vi "WriteINI.vi"(8 "Error In":errorcluster, 11 "ServerINI":T1={"TrackQueues?"=TRUE, "ClientTimeout (s)"=30, "LogPath"=path "C:/Users/jgoebel/Documents/GitHub/AEDashboard/ServerLib/Data/ServerLog.tdms", "ErrorsToIgnore"=[], "OracleData"={"DBname"="", "User"="", "Password"=""}}) -> (0 "Error Out":errorcluster)   [LabVIEW 2017, in "Server.lvlib"]
uses:
  Server.lvlib
  TypeDefs/ServerINI.ctl
  SubLibs/Oracle/OracleData.ctl
  SubLibs/Oracle/Oracle.lvlib
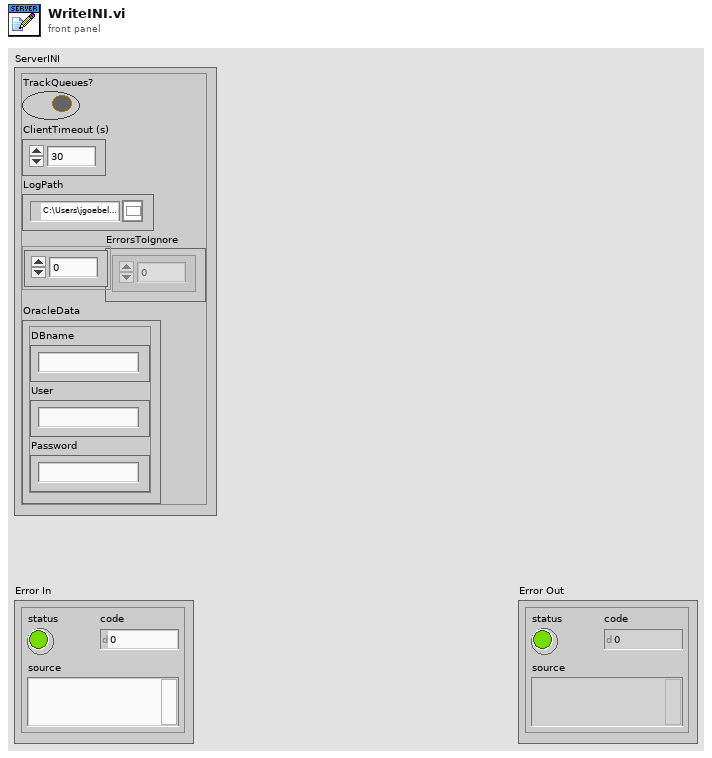
[diagram p1: front panel]
types:
  T1 = typedef "Server.lvlib/ServerINI.ctl" = cluster{"TrackQueues?":bool, "ClientTimeout (s)":u32, "LogPath":path, "ErrorsToIgnore":i32[], "OracleData":T2}
  T2 = typedef "Server.lvlib/Oracle.lvlib/OracleData.ctl" = cluster{"DBname":string, "User":string, "Password":string}
  T3 = enum16{"open", "replace", "create", "open or create", "replace or create", "replace or create with confirmation"}
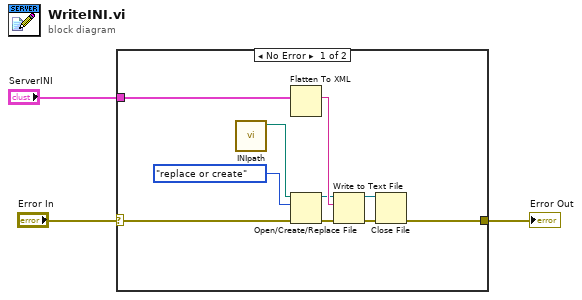
[diagram p0: block diagram]
diagram:
  n1 = case shown="No Error" "Error In" {
    selector: "Error In" -> [w4 w14]
    tunnel: [w6 w14] -> w3
    tunnel: "ServerINI" -> [w5 _]
    frame No Error {
      n2 = call "INIpath.vi"() -> ("appended path"=w13:path)  [unwired: 11 in]
      n3 = Flatten To XML(anything=w5) -> (xml string=w12:string)
      n4 = Open/Create/Replace File(file path (use dialog)=w13, error in=w4, operation (0:open)=T3."replace or create") -> (refnum out=w11:refnum<file>, error out=w7:errorcluster)  [unwired: 3 in, 1 out]
      n5 = Write to Text File(file (use dialog)=w11, text=w12, error in=w7) -> (refnum out=w10:refnum<file>, error out=w9:errorcluster)  [unwired: 1 in, 1 out]
      n6 = Close File(refnum=w10, error in=w9) -> (error out=w6:errorcluster)  [unwired: 1 out]
    }
    frame Error {
    }
  }
  "Error Out" <- w3
